vi "LinearFilter_CutoffFrequency.vi"(11 "TimeConstant":dbl format="%13.5p") -> (3 "Cutoff Freq":dbl format="%13.5p")   [LabVIEW 2019, in "Trajectory_Library.lvlib"]
doc: "Calculate the cutoff frequency from the time constant.\n\nInputs:\n - time Constant - seconds\n\nOutputs:\n - cutoff Frequency - hertz"
uses:
  Trajectory_Library.lvlib
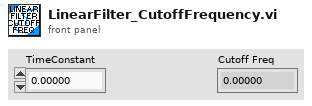
[diagram p1: front panel]
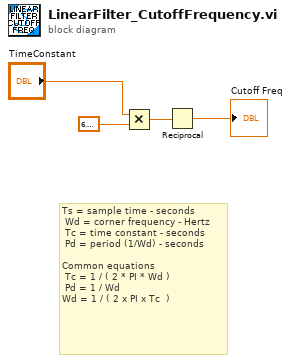
[diagram p0: block diagram]
diagram:
  # "Ts = sample time - seconds\n\tWd = corner frequency - Hertz\n\tTc = time constant - seconds\n\tPd = period (1/Wd) - seconds\n\nCommon equations\n\tTc = 1 / ( 2 * PI * Wd )\n\tPd = 1 / Wd\nWd = 1 / ( 2 x PI x Tc  )"
  n1 = Multiply(x="TimeConstant", y=6.283185307179586) -> (x*y=w3:dbl)
  n2 = Reciprocal(x=w3) -> (1/x=→"Cutoff Freq":dbl)
